vi "Parse JSON Enum Values.vi"(8 "error in":errorcluster, 11 "JSON enum string":string) -> (0 "error out":errorcluster, 2 "sparse enum?":bool, 3 "enum items":string[](array[string]))   [LabVIEW 2021, in "MeasurementClient Editor.lvlib"]
uses:
  MeasurementClient Editor.lvlib
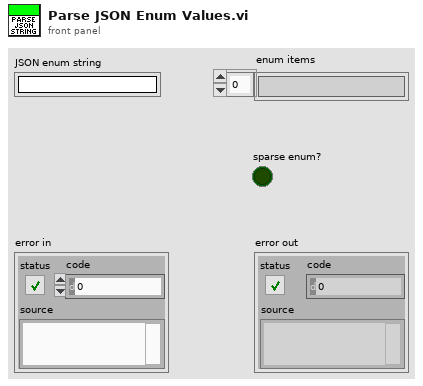
[diagram p1: front panel]
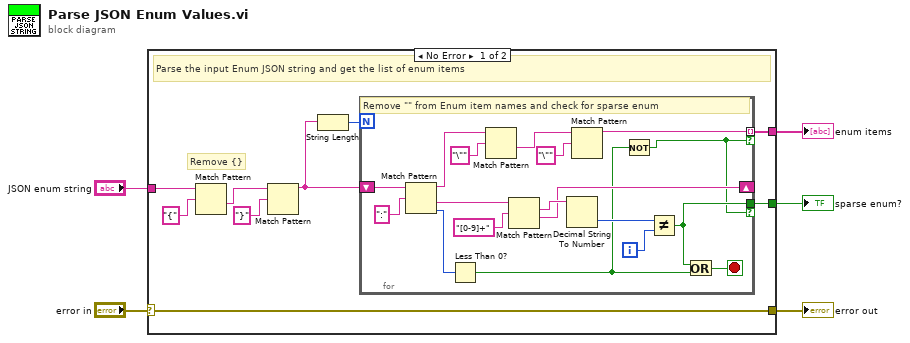
[diagram p0: block diagram]
diagram:
  n1 = case shown="No Error" "error in" {
    selector: "error in" -> [w8 w33]
    tunnel: "JSON enum string" -> [w13 _]
    tunnel: [w10 _] -> w4
    tunnel: [w8 w33] -> w2
    tunnel: [w6 _] -> w1
    frame No Error {
      # "Remove {}"
      # "Parse the input Enum JSON string and get the list of enum items"
      n2 = Match Pattern(string=w13, regular expression="{") -> (after substring=w12:string)  [unwired: 1 in, 3 out]
      n3 = Match Pattern(string=w12, regular expression="}") -> (before substring=w9:string)  [unwired: 1 in, 3 out]
      n4 = String Length(string=w9) -> (length=w7:i32)
      n5 = for {
        N: w7 -> [_]
        shift-right: [w21] -> _
        shift-left: w9 -> [w32]
        tunnel: [w26] -> w10 mode=indexing if=w15
        tunnel: [w16] -> w6 if=w15
        i -> [w19]
        stop <- w18 stop-if-true
        # "Remove \"\" from Enum item names and check for sparse enum"
        n6 = Match Pattern(string=w32, regular expression=":") -> (before substring=w28:string, after substring=w23:string, offset past match=w30:i32)  [unwired: 1 in, 1 out]
        n7 = Less Than 0?(x=w30) -> (x < 0?=w17:bool)
        n8 = Match Pattern(string=w28, regular expression="\"") -> (after substring=w27:string)  [unwired: 1 in, 3 out]
        n9 = Match Pattern(string=w23, regular expression="[0-9]+") -> (match substring=w22:string, after substring=w21:string)  [unwired: 1 in, 2 out]
        n10 = Decimal String To Number(string=w22) -> (number=w20:i32)  [unwired: 2 in, 1 out]
        n11 = Match Pattern(string=w27, regular expression="\"") -> (before substring=w26:string)  [unwired: 1 in, 3 out]
        n12 = Not(x=w17) -> (.not. x?=w15:bool)
        n13 = Not Equal?(x=w20, y=w19) -> (x != y?=w16:bool)
        n14 = Or(x=w16, y=w17) -> (x .or. y?=w18:bool)
      }
    }
    frame Error {
      # "Pass"
    }
  }
  "enum items" <- w4
  "error out" <- w2
  "sparse enum?" <- w1
